vi "fuzzyex Animate Moving Car.vi"(9 "车辆角度（度）":dbl=90.0 format="%.2f", 10 "Y位置":dbl=4.0, 11 "X位置":dbl=1.0) -> (3 "新图片":picture)   [LabVIEW 2018]
doc: "该VI根据位置(X，Y)和角度(Theta)，绘制车辆图。"
uses:
  <vilib>/picture/picture.llb/imagedata.ctl
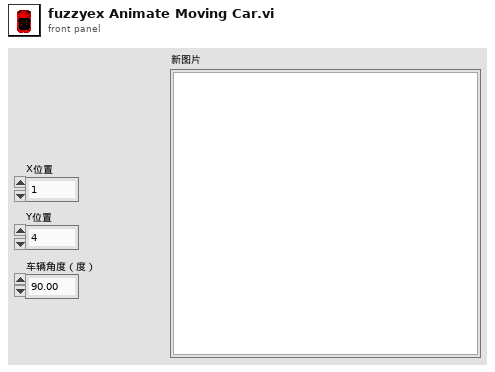
[diagram p1: front panel]
types:
  T1 = typedef "imagedata.ctl" = cluster{"image type":i32, "image depth":i32, "image":u8[], "mask":u8[], "colors":u32[], "Rectangle":cluster{"left":i16, "top":i16, "right":i16, "bottom":i16}}
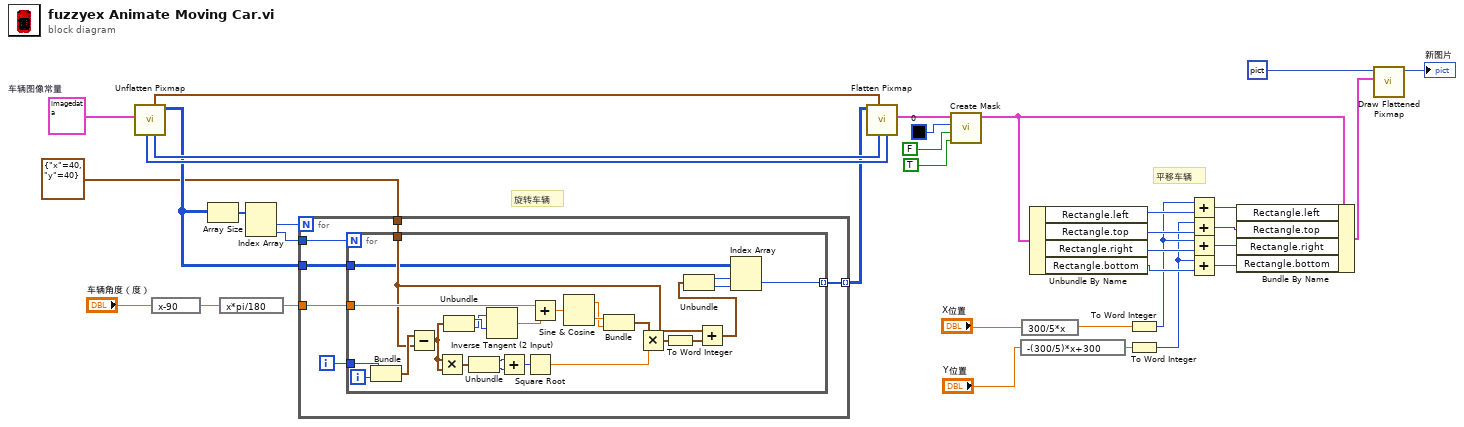
[diagram p0: block diagram]
diagram:
  w32 = T1 {"image type"=0, "image depth"=24, "image"=array[19200 elements], "mask"=[], "colors"=[], "Rectangle"={"left"=0, "top"=0, "right"=80, "bottom"=80}}  # 车辆图像常量
  # "旋转车辆"
  # "平移车辆"
  n1 = call <vilib>:"Unflatten Pixmap.vi"("image data"=w32) -> ("24-bit pixmap"=w24:u32[][], "colors"=w31:u32[], "top left"=w21:cluster{"x":i16, "y":i16}, "mask"=w29:u8[])  [unwired: 7 out]
  n2 = expression code="x-90"("车辆角度（度）") -> (w6:dbl)
  n3 = Array Size(array=w24) -> (size(s)=w35:i32[])
  n4 = expression code="x*pi/180"(w6) -> (w25:dbl)
  n5 = Index Array(array=w35) -> (element #1=w33:i32, element #2=w34:i32)  [unwired: 2 in]
  n6 = for {
    N: w33 -> [_]
    tunnel: w34 -> [w41]
    tunnel: w25 -> [w40]
    tunnel: cluster{"x":i16, "y":i16} {"x"=40, "y"=40} ("Center 2") -> [w39]
    tunnel: w24 -> [w37]
    tunnel: [w36] -> w23 mode=indexing
    i -> [w38]
    n7 = for {
      N: w41 -> [_]
      tunnel: w38 -> [w66]
      tunnel: w40 -> [w56]
      tunnel: w39 -> [w45]
      tunnel: w37 -> [w43]
      tunnel: [w42] -> w36 mode=indexing
      i -> [w44]
      n8 = Bundle(w66, w44) -> (w65:cluster{i32, i32})  [unwired: 1 out]
      n9 = Subtract(x=w65, y=w45) -> (x-y=w60:cluster{i32, i32})
      n10 = Multiply(x=w60, y=w60) -> (x*y=w64:cluster{i32, i32})
      n11 = Unbundle(w60) -> (w59:i32, w58:i32)
      n12 = Unbundle(w64) -> (w63:i32, w62:i32)
      n13 = Inverse Tangent (2 Input)(1:w59, 2:w58) -> (0:w57:dbl)
      n14 = Add(x=w63, y=w62) -> (x+y=w61:i32)
      n15 = Square Root(x=w61) -> (sqrt(x)=w51:dbl)
      n16 = Add(x=w56, y=w57) -> (x+y=w55:dbl)
      n17 = Sine & Cosine(0:w55) -> (1:w53:dbl, 2:w54:dbl)
      n18 = Bundle(w54, w53) -> (w52:cluster{dbl, dbl})  [unwired: 1 out]
      n19 = Multiply(x=w52, y=w51) -> (x*y=w50:cluster{dbl, dbl})
      n20 = To Word Integer(number=w50) -> (16bit integer=w49:cluster{i16, i16})
      n21 = Add(x=w45, y=w49) -> (x+y=w46:cluster{i16, i16})
      n22 = Unbundle(w46) -> (w48:i16, w47:i16)
      n23 = Index Array(array=w43, index (row)=w48, index (col)=w47) -> (element=w42:u32)
    }
  }
  n24 = call <vilib>:"Flatten Pixmap.vi"("mask"=w29, "colors"=w31, "top left"=w21, "24-bit pixmap"=w23) -> ("image data"=w20:T1)  [unwired: 3 in, 4 out]
  n25 = call <vilib>:"Create Mask.vi"("Combine Masks? (F)"=TRUE, "1-Bit Mask Value (T)"=FALSE, "Mask Color (Black)"=u32 0, "image data"=w20) -> ("image data"=w3:T1)  [unwired: 7 out]
  n26 = expression code="-(300/5)*x+300"("Y位置") -> (w8:dbl)
  n27 = expression code="300/5*x"("X位置") -> (w9:dbl)
  n28 = Unbundle By Name(w3) -> ("Rectangle.left"=w19:i16, "Rectangle.top"=w13:i16, "Rectangle.right"=w17:i16, "Rectangle.bottom"=w14:i16)
  n29 = To Word Integer(number=w9) -> (16bit integer=w5:i16)
  n30 = To Word Integer(number=w8) -> (16bit integer=w4:i16)
  n31 = Add(x=w5, y=w19) -> (x+y=w15:i16)
  n32 = Add(x=w4, y=w13) -> (x+y=w11:i16)
  n33 = Add(x=w5, y=w17) -> (x+y=w16:i16)
  n34 = Add(x=w4, y=w14) -> (x+y=w12:i16)
  n35 = Bundle By Name(cluster=w3, "Rectangle.left"=w15, "Rectangle.top"=w11, "Rectangle.right"=w16, "Rectangle.bottom"=w12) -> (w22:T1)
  n36 = call <vilib>:"Draw Flattened Pixmap.vi"("image data"=w22, "picture"=picture data[5B]) -> ("new picture"=→"新图片":picture)  [unwired: 7 out]
